vi "Periodic Tasks.vi"(8 "error in":errorcluster) -> ()   [LabVIEW 2014]
doc: "This VI runs in parallel to other tasks. It can contain as many user-defined periodic loops as you need. These can carry out PID or other sorts of timed response."
uses:
  <vilib>/Rock Robotics/WPI/Solenoid/WPI_SolenoidValue.ctl
  Robot Global Data.vi
  <vilib>/Rock Robotics/WPI/RobotDrive/WPI_RobotDriveGetSetRefNum.vi
  <vilib>/Rock Robotics/WPI/RobotDrive/WPI_RobotDriveMecanumDrive_Cartesian.vi
  <vilib>/Rock Robotics/WPI/Solenoid/WPI_SolenoidSetEnum.vi
  <vilib>/Rock Robotics/Network Tables/SD Read String.vi
  <vilib>/Rock Robotics/Network Tables/SD Read Boolean.vi
  <vilib>/Rock Robotics/Network Tables/SD Write Number.vi
  <vilib>/Rock Robotics/Network Tables/SD Write Boolean.vi
  navX-MXP Library/navX-MXP IMU.lvlib
panel:
  out "AUTO Mode":string
  out "Raw Yaw":dbl
  out "\"Field Centric\" Value":dbl
  out "North":dbl
  out "Level":dbl
  out "Wanted Level":dbl
  out "Left Switch":bool
  out "Right Switch":bool
  out "Bottom Switch":bool
  out "Top Switch":bool
  out "Adjusted Yaw":dbl
  out "Valid?":bool
  # "EDITED: 3/2/15"
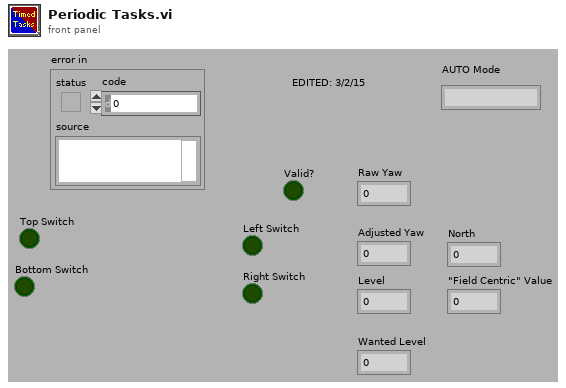
[diagram p1: front panel]
types:
  T1 = typedef "WPI_DigitalInputDevRef.ctl" = cluster{"DevStatus":errorcluster, "DIO Channel":T2, "Controller":T3}
  T2 = typedef "FPGA_DIOChannel.ctl" = enum8{"DIO 0", "DIO 1", "DIO 2", "DIO 3", "DIO 4", "DIO 5", "DIO 6", "DIO 7", "DIO 8", "DIO 9", "DIO MXP 0", "DIO MXP 1", "DIO MXP 2", "DIO MXP 3", "DIO MXP 4", "DIO MXP 5", "DIO MXP 6", "DIO MXP 7", "DIO MXP 8", "DIO MXP 9", "DIO MXP 10", "DIO MXP 11", "DIO MXP 12", "DIO MXP 13", "DIO MXP 14", "DIO MXP 15", "Invalid"}
  T3 = typedef "FPGA_TypedefDigitalModule.ctl" = enum16{"Controller 1"}
  T4 = typedef "navX-MXP IMU.lvlib/navX Device TypeDef.ctl" = cluster{"navX Interface Protocol":T5, "navX Interface Protocol TypeDefs":cluster{"SPIDevRef":T6, "I2CDevRef":T8}, "navX System Information":cluster{"Board Information":T10, "Status":T11, "Offsets":T15}, "navX Common Information":cluster{"Update Rate (4Hz-60Hz)":T16, "refnum name":string, "error":errorcluster}}
  T5 = typedef "navX-MXP IMU.lvlib/navX Interface Protocol.ctl" = enum16{"SPI", "I2C"}
  T6 = typedef "WPI_SPIDevRef.ctl" = cluster{"DevStatus":errorcluster, "Handle":i32, "Controller":T3, "SPI Bus":T7}
  T7 = typedef "spi_bus.ctl" = enum16{"SPI On-Board, CS0", "SPI On-Board, CS1", "SPI On-Board, CS2", "SPI On-Board, CS3", "SPI MXP", "Invalid"}
  T8 = typedef "WPI_I2CDevRef.ctl" = cluster{"DevStatus":errorcluster, "Controller":T3, "Device Address":u8, "Handle":i32, "I2C Bus":T9}
  T9 = typedef "i2c_bus.ctl" = enum16{"I2C On-Board", "I2C MXP", "Invalid"}
  T10 = typedef "navX-MXP IMU.lvlib/navX Board Information.ctl" = cluster{"WhoAmI (50 | 0x32)":u8, "Board Revision":u8, "Firmware Major Version":u8, "Firmware Minor Version":u8}
  T11 = typedef "navX-MXP IMU.lvlib/navX Status Data.ctl" = cluster{"Update Rate Hz":u8, "Accelerometer Full-Scale Range":u8, "Gyro Full-Scale Range":u16, "NAVX_OP_STATUS":T12, "NAVX_CAL_STATUS":T13, "NAVX_SELFTEST_STATUS":u8, "NAVX_SENSOR_STATUS":T14}
  T12 = typedef "navX-MXP IMU.lvlib/navX NAVX_OP_STATUS.ctl" = u8
  T13 = typedef "navX-MXP IMU.lvlib/navX NAVX_CAL_STATUS.ctl" = u8
  T14 = typedef "navX-MXP IMU.lvlib/navX NAVX_SENSOR_STATUS.ctl" = cluster{"MOVING":bool, "YAW_STABLE":bool, "MAG_DISTURBANCE":bool, "ALTITUDE_VALID":bool, "SEALEVEL_PRESS_SET":bool, "FUSED_HEADING_VALID":bool}
  T15 = typedef "navX-MXP IMU.lvlib/navX Offsets Data.ctl" = cluster{"Yaw":dbl, "Quat W":dbl, "Quat X":dbl, "Quat Y":dbl, "Quat Z":dbl}
  T16 = typedef "navX-MXP IMU.lvlib/navX Update Rate.ctl" = u8
  T17 = typedef "navX-MXP IMU.lvlib/navX YPRH Data.ctl" = cluster{"Yaw":dbl, "Pitch":dbl, "Roll":dbl, "Heading":dbl}
  T18 = typedef "WPI_RobotDriveDevRef.ctl" = cluster{"DevStatus":errorcluster, "Motors[]":T19[], "Square Inputs":bool, "Max Output":dbl}
  T19 = typedef "WPI_MotorControlDeviceRef.ctl" = cluster{"DeviceStatus":errorcluster, "Type":T20, "PWM":cluster{"Controller":T3, "PWM Channel":T21, "DeadBand":T22}, "CAN":cluster{"Device Number":u8, "Control Mode":T23, "Semaphore":T24, "Max Vout":dbl, "TalonSRX Control Mode":T25}, "Invert":bool, "TransformRef":T26, "InvTransformRef":T26}
  T20 = typedef "WPI_MotorControlType.ctl" = enum16{"PWM", "CAN", "CANTalonSRX"}
  T21 = typedef "FPGA_DIOPWMChannel.ctl" = enum8{"PWM 0", "PWM 1", "PWM 2", "PWM 3", "PWM 4", "PWM 5", "PWM 6", "PWM 7", "PWM 8", "PWM 9", "PWM MXP 0", "PWM MXP 1", "PWM MXP 2", "PWM MXP 3", "PWM MXP 4", "PWM MXP 5", "PWM MXP 6", "PWM MXP 7", "PWM MXP 8", "PWM MXP 9", "Invalid"}
  T22 = typedef "WPI_PWMDeadband.ctl" = cluster{"Name":string, "maxPositivePwm":i32, "minPositivePwm":i32, "centerPwm":i32, "maxNegativePwm":i32, "minNegativePwm":i32, "angularRange":u16}
  T23 = typedef "WPI_CANJaguar_ControlMode.ctl" = enum8{"Percent VBus", "Current", "Speed", "Position", "Voltage"}
  T24 = typedef "Semaphore RefNum" = refnum<k1>
  T25 = typedef "WPI_CANTalonSRX_APIControlMode.ctl" = enum8{"Percent VBus", "Speed", "Position", "Slave", "Unchanged / Invalid"}
  T26 = typedef "WPI_PWMTransform_ConPane.ctl" = refnum<vi>
  T27 = typedef "WPI_SolenoidDevRef.ctl" = cluster{"DevStatus":errorcluster, "Pneumatics Control Module":u8, "Forward Solenoid Channel":T28, "Reverse Solenoid Channel":T28}
  T28 = typedef "WPI_SolenoidChannel.ctl" = enum8{"Solenoid 0", "Solenoid 1", "Solenoid 2", "Solenoid 3", "Solenoid 4", "Solenoid 5", "Solenoid 6", "Solenoid 7", "Invalid"}
  T29 = typedef "WPI_SolenoidValue.ctl" = enum16{"Off", "On", "Forward", "Reverse"}
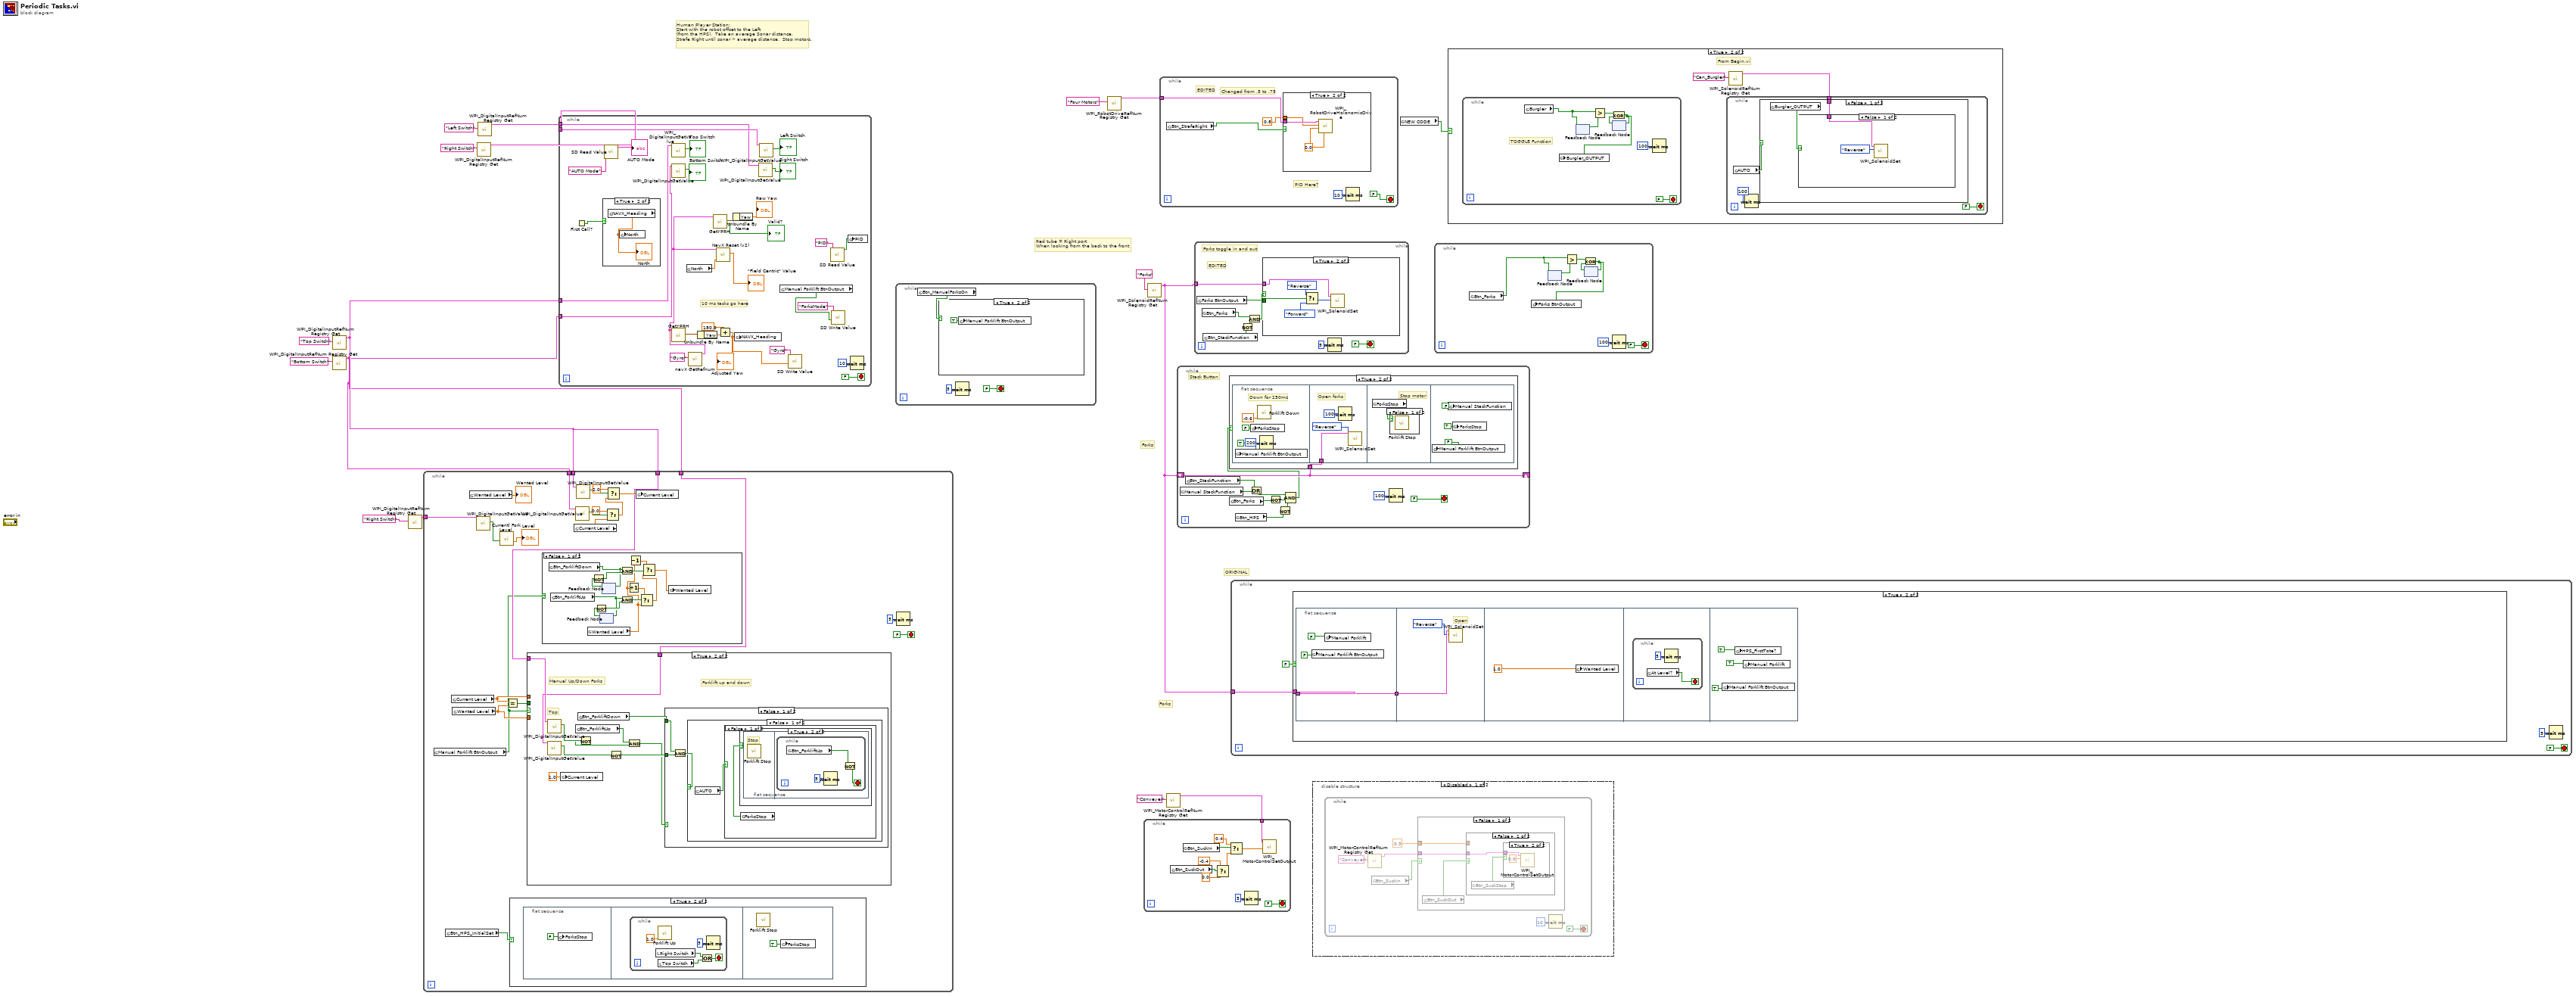
[diagram p0: block diagram]
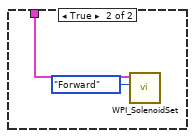
[diagram p3: hidden frame]
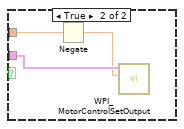
[diagram p6: hidden frame]
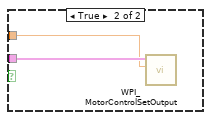
[diagram p7: hidden frame]
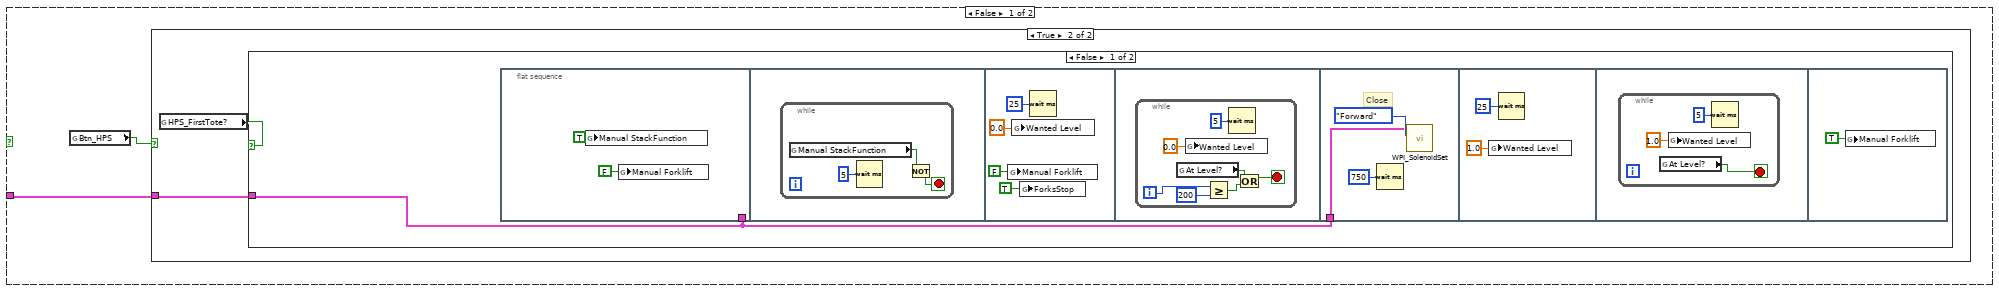
[diagram p9: hidden frame]
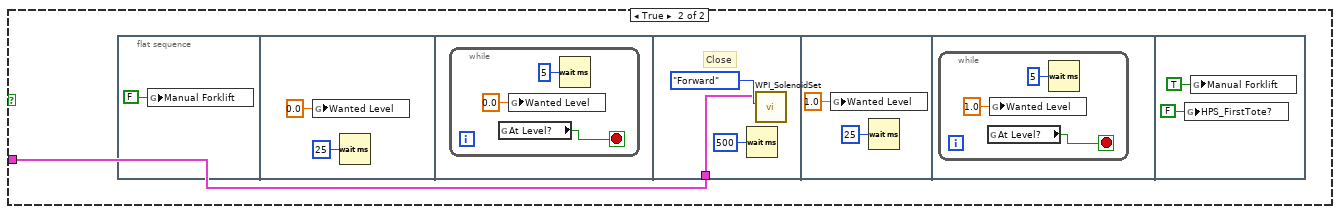
[diagram p11: hidden frame]
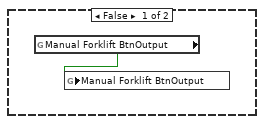
[diagram p13: hidden frame]
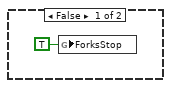
[diagram p14: hidden frame]
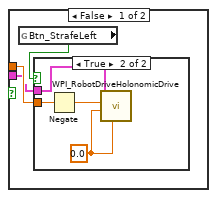
[diagram p17: hidden frame]
diagram:
  # "ORIGINAL"
  # "Forks"
  # "Forks"
  # "Human Player Station:\nStart with the robot offset to the Left\n(from the HPS).  Take an average Sonar distance.\nStrafe Right until sonar > average distance.  Stop motors."
  # "Red tube = Right port\nWhen looking from the back to the front"
  n1 = call <vilib>:"WPI_DigitalInputRefNum Registry Get.vi"("refnum name"="Bottom Switch") -> ("DigitalInputDevRef"=w4:T1)  [unwired: 9 in, 1 out]
  n2 = call <vilib>:"WPI_DigitalInputRefNum Registry Get.vi"("refnum name"="Top Switch") -> ("DigitalInputDevRef"=w5:T1)  [unwired: 9 in, 1 out]
  n3 = call <vilib>:"WPI_DigitalInputRefNum Registry Get.vi"("refnum name"="Right Switch") -> ("DigitalInputDevRef"=w13:T1)  [unwired: 9 in, 1 out]
  n4 = while {
    tunnel: w5 -> [w30]
    tunnel: w4 -> [w29]
    tunnel: w13 -> [w27]
    tunnel: w5 -> [w22]
    tunnel: w4 -> [w21]
    stop <- FALSE stop-if-true
    n5 = global read "Robot Global Data.vi" "Manual Forklift BtnOutput"() -> (w19:bool)
    n6 = global read "Robot Global Data.vi" "Btn_HPS_InitialSet"() -> (w18:bool)
    n7 = global read "Robot Global Data.vi" "Current Level"() -> (w24:dbl)
    n8 = global read "Robot Global Data.vi" "Wanted Level"() -> (w23:dbl)
    n9 = global read "Robot Global Data.vi" "Wanted Level"() -> (→"Wanted Level":dbl)
    n10 = call <vilib>:"WPI_DigitalInputGetValue.vi"("DigitalInputDevRef"=w27) -> ("Value"=w20:bool)  [unwired: 8 in, 2 out]
    n11 = call "Currentl Fork Level.vi"("Right"=w20) -> ("Level"=→"Level":dbl)  [unwired: 10 in]
    n12 = Equal?(x=w24, y=w23) -> (x = y?=w25:bool)
    n13 = case shown="True" w18 {
      frame False {
      }
      frame True {
        n14 = flat-sequence {
          frame #0 {
            n15 = global write "Robot Global Data.vi" "ForksStop"(FALSE ("ForksStop")) -> ()
          }
          frame #1 {
            n16 = while {
              stop <- w42 stop-if-true
              n17 = local read "Right Switch"() -> (w43:bool)
              n18 = call "Forklift Up.vi"("Forklift Up Power"=1.0) -> ()  [unwired: 11 in]
              n19 = local read "Top Switch"() -> (w41:bool)
              n20 = Or(x=w43, y=w41) -> (x .or. y?=w42:bool)
              n21 = Wait (ms)(milliseconds to wait=u32 5) -> ()  [unwired: 1 out]
            }
          }
          frame #2 {
            n22 = call "Forklift Stop.vi"() -> ()  [unwired: 12 in]
            n23 = global write "Robot Global Data.vi" "ForksStop"(TRUE ("ForksStop")) -> ()
          }
        }
      }
    }
    n24 = case shown="True" w19 {
      tunnel: w25 -> [w62 _]
      tunnel: w24 -> [w61 _]
      tunnel: w23 -> [w60 _]
      tunnel: w22 -> [_ w73]
      tunnel: w21 -> [_ w72]
      frame False {
        n25 = case shown="False" w62 {
          tunnel: w61 -> [w64 _]
          tunnel: w60 -> [w63 _]
          frame False {
            n26 = Greater?(x=w64, y=w63) -> (0:w66:bool)
            n27 = case shown="True" w66 {
              frame False {
                n28 = call "Forklift Up.vi"("Forklift Up Power"=1.0) -> ()  [unwired: 11 in]
              }
              frame True {
                n29 = call "Forklift Down.vi"("Forklift Down Speed"=-0.8) -> ()  [unwired: 11 in]
              }
            }
            n30 = global write "Robot Global Data.vi" "At Level?"(FALSE ("ForksStop")) -> ()
          }
          frame True {
            n31 = global read "Robot Global Data.vi" "ForksStop"() -> (w70:bool)
            n32 = case shown="True" w70 {
              frame False {
              }
              frame True {
                n33 = call "Forklift Stop.vi"() -> ()  [unwired: 12 in]
              }
            }
            n34 = global write "Robot Global Data.vi" "At Level?"(TRUE ("ForksStop")) -> ()
          }
        }
      }
      frame True {
        # "Top"
        # "Forklift up and down"
        # "Manual Up/Down Forks"
        n35 = call <vilib>:"WPI_DigitalInputGetValue.vi"("DigitalInputDevRef"=w72) -> ("Value"=w79:bool)  [unwired: 8 in, 2 out]
        n36 = call <vilib>:"WPI_DigitalInputGetValue.vi"("DigitalInputDevRef"=w73) -> ("Value"=w80:bool)  [unwired: 8 in, 2 out]
        n37 = global write "Robot Global Data.vi" "Current Level"(1.0 ("Current Level")) -> ()
        n38 = global read "Robot Global Data.vi" "Btn_ForkliftUp"() -> (w76:bool)
        n39 = global read "Robot Global Data.vi" "Btn_ForkliftDown"() -> (w78:bool)
        n40 = Not(x=w80) -> (.not. x?=w75:bool)
        n41 = Not(x=w79) -> (.not. x?=w77:bool)
        n42 = And(x=w76, y=w75) -> (x .and. y?=w74:bool)
        n43 = case shown="False" w74 {
          tunnel: w78 -> [w81 _]
          tunnel: w77 -> [w82 _]
          frame False {
            n44 = And(x=w81, y=w82) -> (x .and. y?=w83:bool)
            n45 = case shown="False" w83 {
              frame False {
                n46 = global read "Robot Global Data.vi" "AUTO"() -> (w84:bool)
                n47 = case shown="False" w84 {
                  frame False {
                    n48 = global read "Robot Global Data.vi" "ForksStop"() -> (w85:bool)
                    n49 = case shown="True" w85 {
                      frame False {
                      }
                      frame True {
                        n50 = flat-sequence {
                          frame #0 {
                            # "Stop"
                            n51 = call "Forklift Stop.vi"() -> ()  [unwired: 12 in]
                          }
                          frame #1 {
                            n52 = while {
                              stop <- w86 stop-if-true
                              n53 = global read "Robot Global Data.vi" "Btn_ForkliftUp"() -> (w87:bool)
                              n54 = Wait (ms)(milliseconds to wait=u32 5) -> ()  [unwired: 1 out]
                              n55 = Not(x=w87) -> (.not. x?=w86:bool)
                            }
                          }
                        }
                      }
                    }
                  }
                  frame True {
                  }
                }
              }
              frame True {
                # "Down"
                n56 = call "Forklift Down.vi"("Forklift Down Speed"=-0.8) -> ()  [unwired: 11 in]
              }
            }
          }
          frame True {
            # "Up"
            n57 = call "Forklift Up.vi"("Forklift Up Power"=1.0) -> ()  [unwired: 11 in]
          }
        }
      }
    }
    n58 = case shown="False" w19 {
      frame False {
        n59 = global read "Robot Global Data.vi" "Btn_ForkliftDown"() -> (w54:bool)
        n60 = global read "Robot Global Data.vi" "Btn_ForkliftUp"() -> (w58:bool)
        n61 = global read "Robot Global Data.vi" "Wanted Level"() -> (w47:dbl)
        n62 = feedback #1() -> (w57:bool)  [unwired: 1 in]
        n63 = Not(x=w57) -> (.not. x?=w59:bool)
        n64 = feedback-in #1(w58) -> ()
        n65 = feedback #2() -> (w55:bool)  [unwired: 1 in]
        n66 = Not(x=w55) -> (.not. x?=w56:bool)
        n67 = feedback-in #2(w54) -> ()
        n68 = And(x=w54, y=w56) -> (x .and. y?=w53:bool)
        n69 = And(x=w58, y=w59) -> (x .and. y?=w52:bool)
        n70 = Increment(x=w47) -> (x+1=w50:dbl)
        n71 = Decrement(x=w47) -> (x-1=w48:dbl)
        n72 = Select(t=w50, s=w52, f=w47) -> (s? t:f=w51:dbl)
        n73 = Select(t=w48, s=w53, f=w51) -> (s? t:f=w49:dbl)
        n74 = global write "Robot Global Data.vi" "Wanted Level"(w49) -> ()
      }
      frame True {
      }
    }
    n75 = global read "Robot Global Data.vi" "Current Level"() -> (w37:dbl)
    n76 = call <vilib>:"WPI_DigitalInputGetValue.vi"("DigitalInputDevRef"=w29) -> ("Value"=w32:bool)  [unwired: 8 in, 2 out]
    n77 = call <vilib>:"WPI_DigitalInputGetValue.vi"("DigitalInputDevRef"=w30) -> ("Value"=w31:bool)  [unwired: 8 in, 2 out]
    n78 = Select(t=0.0, s=w32, f=w37) -> (s? t:f=w36:dbl)
    n79 = Select(t=2.0, s=w31, f=w36) -> (s? t:f=w35:dbl)
    n80 = global write "Robot Global Data.vi" "Current Level"(w35) -> ()
    n81 = Wait (ms)(milliseconds to wait=u32 5) -> ()  [unwired: 1 out]
  }
  n82 = call <vilib>:"WPI_DigitalInputRefNum Registry Get.vi"("refnum name"="Right Switch") -> ("DigitalInputDevRef"=w6:T1)  [unwired: 9 in, 1 out]
  n83 = call <vilib>:"WPI_DigitalInputRefNum Registry Get.vi"("refnum name"="Left Switch") -> ("DigitalInputDevRef"=w7:T1)  [unwired: 9 in, 1 out]
  n84 = while {
    tunnel: w5 -> [w117]
    tunnel: w4 -> [w116]
    tunnel: w7 -> [w111]
    tunnel: w6 -> [w110]
    stop <- FALSE stop-if-true
    # "10 ms tasks go here"
    n85 = First Call?() -> (First Call?: T/F=w100:bool)
    n86 = case shown="True" w100 {
      frame False {
      }
      frame True {
        n87 = global read "Robot Global Data.vi" "NAVX_Heading"() -> (w120:dbl)
        "North" <- w120
        n88 = global write "Robot Global Data.vi" "North"(w120) -> ()
      }
    }
    n89 = call-poly <vilib>:"SD Read Value.vi"("Name"="AUTO Mode") -> ("String"=→"AUTO Mode":string)  [unwired: 8 in, 2 out]
    n90 = call <vilib>:"WPI_DigitalInputGetValue.vi"("DigitalInputDevRef"=w116) -> ("Value"=→"Bottom Switch":bool)  [unwired: 8 in, 2 out]
    n91 = call <vilib>:"WPI_DigitalInputGetValue.vi"("DigitalInputDevRef"=w117) -> ("Value"=→"Top Switch":bool)  [unwired: 8 in, 2 out]
    n92 = global read "Robot Global Data.vi" "North"() -> (w99:dbl)
    n93 = call "navX GetRefnum.vi"("refnum name"="Gyro") -> ("navX Device TypeDef"=w101:T4)  [unwired: 9 in, 1 out]
    n94 = call "GetYPRH.vi"("navX Device TypeDef"=w101) -> ("YPRH"=w109:T17)  [unwired: 8 in, 2 out]
    n95 = Unbundle By Name(w109) -> ("Yaw"=w108:dbl)
    n96 = call "GetYPRH.vi"("navX Device TypeDef"=w101) -> ("Valid?"=→"Valid?":bool, "YPRH"=w104:T17)  [unwired: 8 in, 1 out]
    n97 = call "NavX Reset (v2).vi"("North In"=w99, "navX Device TypeDef"=w101) -> ("Output Angle"=→"\"Field Centric\" Value":dbl)  [unwired: 9 in]
    n98 = Add(x=180.0, y=w108) -> (x+y=w92:dbl)
    "Adjusted Yaw" <- w92
    n99 = Unbundle By Name(w104) -> ("Yaw"=→"Raw Yaw":dbl)
    n100 = global write "Robot Global Data.vi" "NAVX_Heading"(w92) -> ()
    n101 = call <vilib>:"WPI_DigitalInputGetValue.vi"("DigitalInputDevRef"=w110) -> ("Value"=→"Right Switch":bool)  [unwired: 8 in, 2 out]
    n102 = call <vilib>:"WPI_DigitalInputGetValue.vi"("DigitalInputDevRef"=w111) -> ("Value"=→"Left Switch":bool)  [unwired: 8 in, 2 out]
    n103 = global read "Robot Global Data.vi" "Manual Forklift BtnOutput"() -> (w95:bool)
    n104 = call-poly <vilib>:"SD Write Value.vi"("Numeric"=w92, "Name"="Gyro") -> ()  [unwired: 8 in, 2 out]
    n105 = call-poly <vilib>:"SD Read Value.vi"("Name"="PID") -> ("Boolean"=w93:bool)  [unwired: 8 in, 2 out]
    n106 = call-poly <vilib>:"SD Write Value.vi"("Boolean"=w95, "Name"="ForksMode") -> ()  [unwired: 8 in, 2 out]
    n107 = global write "Robot Global Data.vi" "PID"(w93) -> ()
    n108 = Wait (ms)(milliseconds to wait=u32 10) -> ()  [unwired: 1 out]
  }
  n109 = while {
    stop <- FALSE stop-if-true
    n110 = global read "Robot Global Data.vi" "Btn_ManualForksOn"() -> (w121:bool)
    n111 = case shown="True" w121 {
      frame False {
        n112 = global read "Robot Global Data.vi" "Manual Forklift BtnOutput"() -> (w124:bool)
        n113 = global write "Robot Global Data.vi" "Manual Forklift BtnOutput"(w124) -> ()
      }
      frame True {
        n114 = global write "Robot Global Data.vi" "Manual Forklift BtnOutput"(TRUE ("Btn_ManualDriveToggle")) -> ()
      }
    }
    n115 = Wait (ms)(milliseconds to wait=u32 5) -> ()  [unwired: 1 out]
  }
  n116 = call <vilib>:"WPI_RobotDriveRefNum Registry Get.vi"("refnum name"="Four Motors") -> ("RobotDriveDevRef"=w11:T18)  [unwired: 9 in, 1 out]
  n117 = call <vilib>:"WPI_SolenoidRefNum Registry Get.vi"("refnum name"="Forks") -> ("SolenoidDevRef"=w15:T27)  [unwired: 9 in, 1 out]
  n118 = while {
    tunnel: w11 -> [w128]
    stop <- FALSE stop-if-true
    # "Changed from .5 to .75"
    # "EDITED"
    # "PID Here?"
    n119 = global read "Robot Global Data.vi" "Btn_StrafeRight"() -> (w126:bool)
    n120 = case shown="True" w126 {
      tunnel: w128 -> [w131 w140]
      tunnel: 0.8 ("t") -> [w132 w139]
      frame False {
        n121 = global read "Robot Global Data.vi" "Btn_StrafeLeft"() -> (w133:bool)
        n122 = case shown="True" w133 {
          tunnel: w132 -> [_ w137]
          tunnel: w131 -> [_ w135]
          frame False {
          }
          frame True {
            w134 = 0.0 ("Rotation")
            n123 = Negate(x=w137) -> (-x=w136:dbl)
            n124 = call-poly <vilib>:"WPI_RobotDriveHolonomicDrive.vi"("Rotation"=w134, "Y"=w134, "X"=w136, "RobotDriveDevRef"=w135) -> ()  [unwired: 5 in, 3 out]
          }
        }
      }
      frame True {
        w138 = 0.0 ("Rotation")
        n125 = call-poly <vilib>:"WPI_RobotDriveHolonomicDrive.vi"("Rotation"=w138, "Y"=w138, "X"=w139, "RobotDriveDevRef"=w140) -> ()  [unwired: 5 in, 3 out]
      }
    }
    n126 = Wait (ms)(milliseconds to wait=u32 10) -> ()  [unwired: 1 out]
  }
  n127 = call <vilib>:"WPI_MotorControlRefNum Registry Get.vi"("refnum name"="Conveyer") -> ("MotorControlDevRef"=w2:T19)  [unwired: 9 in, 1 out]
  n128 = while {
    tunnel: w2 -> [w141]
    stop <- FALSE stop-if-true
    n129 = global read "Robot Global Data.vi" "Btn_SuckOut"() -> (w148:bool)
    n130 = global read "Robot Global Data.vi" "Btn_SuckIn"() -> (w150:bool)
    n131 = Select(t=-0.4, s=w148, f=0.0) -> (s? t:f=w149:dbl)
    n132 = Select(t=0.4, s=w150, f=w149) -> (s? t:f=w144:dbl)
    n133 = Wait (ms)(milliseconds to wait=u32 5) -> ()  [unwired: 1 out]
    n134 = call <vilib>:"WPI_MotorControlSetOutput.vi"("Output"=w144, "MotorControlDevRef"=w141) -> ()  [unwired: 7 in, 3 out]
  }
  n135 = while {
    shift-right: [w159] -> _
    shift-left: w15 -> [w159]
    stop <- FALSE stop-if-true
    # "Stack Button"
    n136 = global read "Robot Global Data.vi" "Manual StackFunction"() -> (w151:bool)
    n137 = global read "Robot Global Data.vi" "Btn_StackFunction"() -> (w158:bool)
    n138 = global read "Robot Global Data.vi" "Btn_Forks"() -> (w157:bool)
    n139 = global read "Robot Global Data.vi" "Btn_HPS"() -> (w154:bool)
    n140 = Or(x=w158, y=w151) -> (x .or. y?=w152:bool)
    n141 = Not(x=w157) -> (.not. x?=w156:bool)
    n142 = Not(x=w154) -> (.not. x?=w153:bool)
    n143 = Compound Arithmetic op=AND(w152, w156, w153) -> (w155:bool)
    n144 = case shown="True" w155 {
      tunnel: w159 -> [_ w163]
      frame False {
        n145 = global write "Robot Global Data.vi" "ForksStop"(TRUE ("ForksStop")) -> ()
      }
      frame True {
        n146 = flat-sequence {
          tunnel: w163 -> [w168]
          frame #0 {
            # "Down for 250ms"
            n147 = global write "Robot Global Data.vi" "Manual Forklift BtnOutput"(TRUE ("Manual Forklift")) -> ()
            n148 = global write "Robot Global Data.vi" "ForksStop"(FALSE ("ForksStop")) -> ()
            n149 = call "Forklift Down.vi"("Forklift Down Speed"=-0.6) -> ()  [unwired: 11 in]
            n150 = Wait (ms)(milliseconds to wait=u32 200) -> ()  [unwired: 1 out]
          }
          frame #1 {
            # "Open forks"
            n151 = Wait (ms)(milliseconds to wait=u32 100) -> ()  [unwired: 1 out]
            n152 = call-poly <vilib>:"WPI_SolenoidSet.vi"("Value"=WPI_SolenoidValue."Reverse", "SolenoidDevRef"=w168) -> ()  [unwired: 8 in, 2 out]
          }
          frame #2 {
            # "Stop motor"
            n153 = global read "Robot Global Data.vi" "ForksStop"() -> (w171:bool)
            n154 = case shown="False" w171 {
              frame False {
                n155 = call "Forklift Stop.vi"() -> ()  [unwired: 12 in]
              }
              frame True {
              }
            }
          }
          frame #3 {
            n156 = global write "Robot Global Data.vi" "Manual Forklift BtnOutput"(FALSE ("ForksStop")) -> ()
            n157 = global write "Robot Global Data.vi" "Manual StackFunction"(FALSE ("Btn_StackFunction")) -> ()
            n158 = global write "Robot Global Data.vi" "ForksStop"(TRUE ("ForksStop")) -> ()
          }
        }
      }
    }
    n159 = Wait (ms)(milliseconds to wait=u32 100) -> ()  [unwired: 1 out]
  }
  n160 = while {
    tunnel: w15 -> [w175]
    stop <- FALSE stop-if-true
    # "EDITED"
    # "Forks toggle in and out"
    n161 = global read "Robot Global Data.vi" "Forks BtnOutput"() -> (w177:bool)
    n162 = global read "Robot Global Data.vi" "Btn_Forks"() -> (w176:bool)
    n163 = global read "Robot Global Data.vi" "Btn_StackFunction"() -> (w180:bool)
    n164 = Not(x=w180) -> (.not. x?=w179:bool)
    n165 = And(x=w176, y=w179) -> (x .and. y?=w178:bool)
    n166 = case shown="True" w178 {
      tunnel: w175 -> [_ w183]
      tunnel: w177 -> [_ w186]
      frame False {
      }
      frame True {
        n167 = Select(t=WPI_SolenoidValue."Reverse", s=w186, f=WPI_SolenoidValue."Forward" ("Value")) -> (s? t:f=w185:T29)
        n168 = call-poly <vilib>:"WPI_SolenoidSet.vi"("Value"=w185, "SolenoidDevRef"=w183) -> ()  [unwired: 8 in, 2 out]
      }
    }
    n169 = Wait (ms)(milliseconds to wait=u32 5) -> ()  [unwired: 1 out]
  }
  n170 = while {
    tunnel: w15 -> [w189]
    stop <- FALSE stop-if-true
    n171 = case shown="True" FALSE {
      tunnel: w189 -> [w192 w240]
      frame False {
        n172 = global read "Robot Global Data.vi" "Btn_HPS"() -> (w193:bool)
        n173 = case shown="True" w193 {
          tunnel: w192 -> [_ w194]
          frame False {
          }
          frame True {
            n174 = global read "Robot Global Data.vi" "HPS_FirstTote?"() -> (w195:bool)
            n175 = case shown="False" w195 {
              tunnel: w194 -> [w196 w222]
              frame False {
                n176 = flat-sequence {
                  tunnel: w196 -> [_]
                  tunnel: w196 -> [w213]
                  frame #0 {
                    n177 = global write "Robot Global Data.vi" "Manual StackFunction"(TRUE ("Btn_StackFunction")) -> ()
                    n178 = global write "Robot Global Data.vi" "Manual Forklift"(FALSE ("HPS_FirstTote?")) -> ()
                  }
                  frame #1 {
                    n179 = while {
                      stop <- w199 stop-if-true
                      n180 = global read "Robot Global Data.vi" "Manual StackFunction"() -> (w201:bool)
                      n181 = Wait (ms)(milliseconds to wait=u32 5) -> ()  [unwired: 1 out]
                      n182 = Not(x=w201) -> (.not. x?=w199:bool)
                    }
                  }
                  frame #2 {
                    n183 = global write "Robot Global Data.vi" "Manual Forklift"(FALSE ("HPS_FirstTote?")) -> ()
                    n184 = global write "Robot Global Data.vi" "Wanted Level"(0.0 ("Wanted Level")) -> ()
                    n185 = global write "Robot Global Data.vi" "ForksStop"(TRUE ("ForksStop")) -> ()
                    n186 = Wait (ms)(milliseconds to wait=u32 25) -> ()  [unwired: 1 out]
                  }
                  frame #3 {
                    n187 = while {
                      i -> [w209]
                      stop <- w207 stop-if-true
                      n188 = global read "Robot Global Data.vi" "At Level?"() -> (w212:bool)
                      n189 = global write "Robot Global Data.vi" "Wanted Level"(0.0 ("Wanted Level")) -> ()
                      n190 = Greater Or Equal?(x=w209, y=200) -> (x >= y?=w206:bool)
                      n191 = Wait (ms)(milliseconds to wait=u32 5) -> ()  [unwired: 1 out]
                      n192 = Or(x=w212, y=w206) -> (x .or. y?=w207:bool)
                    }
                  }
                  frame #4 {
                    # "Close"
                    n193 = Wait (ms)(milliseconds to wait=u32 750) -> ()  [unwired: 1 out]
                    n194 = call-poly <vilib>:"WPI_SolenoidSet.vi"("Value"=WPI_SolenoidValue."Forward", "SolenoidDevRef"=w213) -> ()  [unwired: 8 in, 2 out]
                  }
                  frame #5 {
                    n195 = global write "Robot Global Data.vi" "Wanted Level"(1.0 ("Wanted Level")) -> ()
                    n196 = Wait (ms)(milliseconds to wait=u32 25) -> ()  [unwired: 1 out]
                  }
                  frame #6 {
                    n197 = while {
                      stop <- w220 stop-if-true
                      n198 = global read "Robot Global Data.vi" "At Level?"() -> (w220:bool)
                      n199 = global write "Robot Global Data.vi" "Wanted Level"(1.0 ("Wanted Level")) -> ()
                      n200 = Wait (ms)(milliseconds to wait=u32 5) -> ()  [unwired: 1 out]
                    }
                  }
                  frame #7 {
                    n201 = global write "Robot Global Data.vi" "Manual Forklift"(TRUE ("HPS_FirstTote?")) -> ()
                  }
                }
              }
              frame True {
                n202 = flat-sequence {
                  tunnel: w222 -> [w230]
                  frame #0 {
                    n203 = global write "Robot Global Data.vi" "Manual Forklift"(FALSE ("Manual Forklift")) -> ()
                  }
                  frame #1 {
                    n204 = global write "Robot Global Data.vi" "Wanted Level"(0.0 ("Wanted Level")) -> ()
                    n205 = Wait (ms)(milliseconds to wait=u32 25) -> ()  [unwired: 1 out]
                  }
                  frame #2 {
                    n206 = while {
                      stop <- w228 stop-if-true
                      n207 = global read "Robot Global Data.vi" "At Level?"() -> (w228:bool)
                      n208 = global write "Robot Global Data.vi" "Wanted Level"(0.0 ("Wanted Level")) -> ()
                      n209 = Wait (ms)(milliseconds to wait=u32 5) -> ()  [unwired: 1 out]
                    }
                  }
                  frame #3 {
                    # "Close"
                    n210 = Wait (ms)(milliseconds to wait=u32 500) -> ()  [unwired: 1 out]
                    n211 = call-poly <vilib>:"WPI_SolenoidSet.vi"("Value"=WPI_SolenoidValue."Forward", "SolenoidDevRef"=w230) -> ()  [unwired: 8 in, 2 out]
                  }
                  frame #4 {
                    n212 = global write "Robot Global Data.vi" "Wanted Level"(1.0 ("Wanted Level")) -> ()
                    n213 = Wait (ms)(milliseconds to wait=u32 25) -> ()  [unwired: 1 out]
                  }
                  frame #5 {
                    n214 = while {
                      stop <- w236 stop-if-true
                      n215 = global read "Robot Global Data.vi" "At Level?"() -> (w236:bool)
                      n216 = global write "Robot Global Data.vi" "Wanted Level"(1.0 ("Wanted Level")) -> ()
                      n217 = Wait (ms)(milliseconds to wait=u32 5) -> ()  [unwired: 1 out]
                    }
                  }
                  frame #6 {
                    n218 = global write "Robot Global Data.vi" "HPS_FirstTote?"(FALSE ("HPS_FirstTote?")) -> ()
                    n219 = global write "Robot Global Data.vi" "Manual Forklift"(TRUE ("Manual Forklift")) -> ()
                  }
                }
              }
            }
          }
        }
      }
      frame True {
        n220 = flat-sequence {
          tunnel: w240 -> [w243]
          tunnel: [w243] -> w239
          tunnel: w239 -> [w245]
          frame #0 {
            n221 = global write "Robot Global Data.vi" "Manual Forklift BtnOutput"(FALSE ("HPS_FirstTote?")) -> ()
            n222 = global write "Robot Global Data.vi" "Manual Forklift"(FALSE ("HPS_FirstTote?")) -> ()
          }
          frame #1 {
            # "Open"
            n223 = call-poly <vilib>:"WPI_SolenoidSet.vi"("Value"=WPI_SolenoidValue."Reverse", "SolenoidDevRef"=w245) -> ()  [unwired: 8 in, 2 out]
          }
          frame #2 {
            n224 = global write "Robot Global Data.vi" "Wanted Level"(1.0 ("Wanted Level")) -> ()
          }
          frame #3 {
            n225 = while {
              stop <- w248 stop-if-true
              n226 = global read "Robot Global Data.vi" "At Level?"() -> (w248:bool)
              n227 = Wait (ms)(milliseconds to wait=u32 5) -> ()  [unwired: 1 out]
            }
          }
          frame #4 {
            n228 = global write "Robot Global Data.vi" "Manual Forklift BtnOutput"(TRUE ("HPS_FirstTote?")) -> ()
            n229 = global write "Robot Global Data.vi" "HPS_FirstTote?"(TRUE ("HPS_FirstTote?")) -> ()
            n230 = global write "Robot Global Data.vi" "Manual Forklift"(TRUE ("HPS_FirstTote?")) -> ()
          }
        }
      }
    }
    n231 = Wait (ms)(milliseconds to wait=u32 5) -> ()  [unwired: 1 out]
  }
  n232 = disable-structure shown="Disabled" {
    frame Disabled {
      n233 = while {
        stop <- FALSE stop-if-true
        n234 = call <vilib>:"WPI_MotorControlRefNum Registry Get.vi"("refnum name"="Conveyer") -> ("MotorControlDevRef"=w256:T19)  [unwired: 9 in, 1 out]
        n235 = global read "Robot Global Data.vi" "Btn_SuckIn"() -> (w255:bool)
        n236 = case shown="False" w255 {
          tunnel: w256 -> [w260 w269]
          tunnel: 0.3 ("t") -> [w258 w268]
          frame False {
            n237 = global read "Robot Global Data.vi" "Btn_SuckOut"() -> (w259:bool)
            n238 = case shown="False" w259 {
              tunnel: w260 -> [w261 w267]
              tunnel: w258 -> [_ w266]
              frame False {
                n239 = global read "Robot Global Data.vi" "Btn_SuckStop"() -> (w262:bool)
                n240 = case shown="True" w262 {
                  tunnel: w261 -> [_ w264]
                  frame False {
                  }
                  frame True {
                    n241 = call <vilib>:"WPI_MotorControlSetOutput.vi"("Output"=0.0, "MotorControlDevRef"=w264) -> ()  [unwired: 7 in, 3 out]
                  }
                }
              }
              frame True {
                n242 = Negate(x=w266) -> (-x=w265:dbl)
                n243 = call <vilib>:"WPI_MotorControlSetOutput.vi"("Output"=w265, "MotorControlDevRef"=w267) -> ()  [unwired: 7 in, 3 out]
              }
            }
          }
          frame True {
            n244 = call <vilib>:"WPI_MotorControlSetOutput.vi"("Output"=w268, "MotorControlDevRef"=w269) -> ()  [unwired: 7 in, 3 out]
          }
        }
        n245 = Wait (ms)(milliseconds to wait=u32 10) -> ()  [unwired: 1 out]
      }
    }
    frame Enabled {
    }
  }
  n246 = global read "Robot Global Data.vi" "NEW CODE"() -> (w1:bool)
  n247 = while {
    stop <- FALSE stop-if-true
    n248 = global read "Robot Global Data.vi" "Btn_Forks"() -> (w271:bool)
    n249 = feedback #3() -> (w274:bool)  [unwired: 1 out]
    n250 = feedback-in #3(w271) -> ()
    n251 = Greater?(x=w271, y=w274) -> (0:w273:bool)
    n252 = feedback #4() -> (w272:bool)  [unwired: 1 out]
    n253 = Exclusive Or(1:w272, 2:w273) -> (0:w270:bool)
    n254 = global write "Robot Global Data.vi" "Forks BtnOutput"(w270) -> ()
    n255 = feedback-in #4(w270) -> ()
    n256 = Wait (ms)(milliseconds to wait=u32 100) -> ()  [unwired: 1 out]
  }
  n257 = case shown="True" w1 {
    frame False {
    }
    frame True {
      # "From Begin.vi"
      n258 = while {
        stop <- FALSE stop-if-true
        # "TOGGLE Function"
        n259 = global read "Robot Global Data.vi" "Burgler"() -> (w290:bool)
        n260 = feedback #5() -> (w293:bool)  [unwired: 1 out]
        n261 = feedback-in #5(w290) -> ()
        n262 = Greater?(x=w290, y=w293) -> (0:w292:bool)
        n263 = feedback #6() -> (w291:bool)  [unwired: 1 out]
        n264 = Exclusive Or(1:w291, 2:w292) -> (0:w289:bool)
        n265 = global write "Robot Global Data.vi" "Burgler_OUTPUT"(w289) -> ()
        n266 = feedback-in #6(w289) -> ()
        n267 = Wait (ms)(milliseconds to wait=u32 100) -> ()  [unwired: 1 out]
      }
      n268 = call <vilib>:"WPI_SolenoidRefNum Registry Get.vi"("refnum name"="Can_Burgler") -> ("SolenoidDevRef"=w277:T27)  [unwired: 9 in, 1 out]
      n269 = while {
        tunnel: w277 -> [w281]
        stop <- FALSE stop-if-true
        n270 = global read "Robot Global Data.vi" "AUTO"() -> (w279:bool)
        n271 = Wait (ms)(milliseconds to wait=u32 100) -> ()  [unwired: 1 out]
        n272 = case shown="False" w279 {
          tunnel: w281 -> [w284 _]
          frame False {
            n273 = global read "Robot Global Data.vi" "Burgler_OUTPUT"() -> (w283:bool)
            n274 = case shown="False" w283 {
              tunnel: w284 -> [w285 w288]
              frame False {
                n275 = call-poly <vilib>:"WPI_SolenoidSet.vi"("Value"=WPI_SolenoidValue."Reverse", "SolenoidDevRef"=w285) -> ()  [unwired: 8 in, 2 out]
              }
              frame True {
                n276 = call-poly <vilib>:"WPI_SolenoidSet.vi"("Value"=WPI_SolenoidValue."Forward", "SolenoidDevRef"=w288) -> ()  [unwired: 8 in, 2 out]
              }
            }
          }
          frame True {
          }
        }
      }
    }
  }
